vi "Com_SECS Equipment _Initialize.vi"(8 "error in":errorcluster, 10 "Timeout":i32=1000, 11 "Connection Setting":T2) -> (0 "error out":errorcluster, 3 "Buffer Data":T1)   [LabVIEW 2018]
uses:
  Data Def/Com_SECS Equipment _Connection Setting.ctl
  Data Def/Com_SECS Equipment _Buffer Data.ctl
  Data Def/Com_SECS Equipment _Timeout Setting.ctl
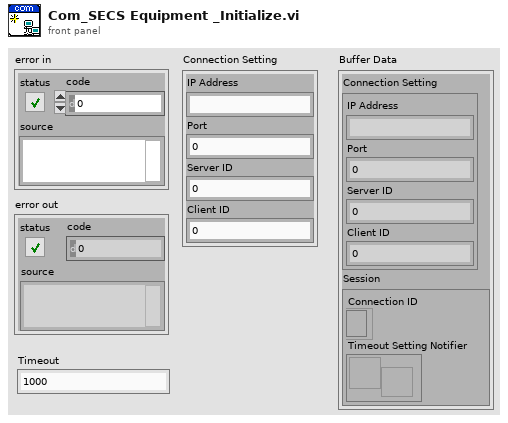
[diagram p1: front panel]
types:
  T1 = typedef "Com_SECS Equipment _Buffer Data.ctl" = cluster{"Connection Setting":T2, "Session":cluster{"Connection ID":refnum<k5>, "Timeout Setting Notifier":refnum<notifier>}}
  T2 = typedef "Com_SECS Equipment _Connection Setting.ctl" = cluster{"IP Address":string, "Port":u16, "Server ID":u16, "Client ID":u16}
  T3 = typedef "Com_SECS Equipment _Timeout Setting.ctl" = cluster{"T3(Reply Timeout)":dbl, "T5(Separation Timeout)":dbl, "T6(Control Timeout)":dbl, "T7(Not Selected Timeout)":dbl, "T8(Inter-Character Timeout)":dbl}
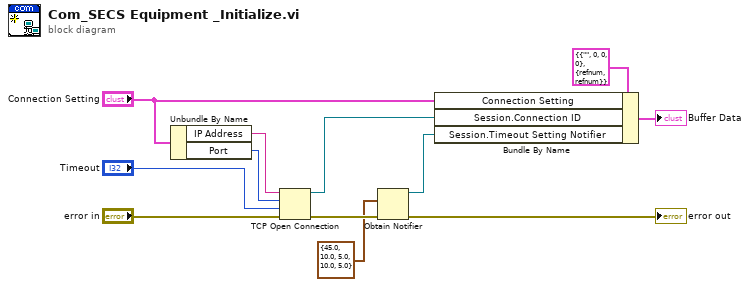
[diagram p0: block diagram]
diagram:
  n1 = Unbundle By Name("Connection Setting") -> ("IP Address"=w11:string, "Port"=w12:u16)
  n2 = TCP Open Connection(address=w11, remote port or service name=w12, timeout ms (60000)="Timeout", error in (no error)="error in") -> (connection ID=w6:refnum<k5>, error out=w4:errorcluster)  [unwired: 1 in]
  n3 = Obtain Notifier(notification data type=T3 {"T3(Reply Timeout)"=45.0, "T5(Separation Timeout)"=10.0, "T6(Control Timeout)"=5.0, "T7(Not Selected Timeout)"=10.0, "T8(Inter-Character Timeout)"=5.0} ("Timeout Setting"), error in (no error)=w4) -> (notifier out=w2:refnum<notifier>, error out=→"error out":errorcluster)  [unwired: 2 in, 1 out]
  n4 = Bundle By Name(cluster=T1 {"Connection Setting"={"IP Address"="", "Port"=0, "Server ID"=0, "Client ID"=0}, "Session"={"Connection ID"=refnum, "Timeout Setting Notifier"=refnum}} ("Buffer Data"), "Connection Setting"="Connection Setting", "Session.Connection ID"=w6, "Session.Timeout Setting Notifier"=w2) -> (→"Buffer Data":T1)
